vi "PitchCalc.vi"(10 "Previous Pitch Value":dbl, 11 "Pitch Control":dbl) -> (2 "New Pitch Value":dbl, 3 "Adjustment to be made":dbl)   [LabVIEW 2014, in "lv-attitudecontrol.lvlib"]
uses:
  lv-attitudecontrol.lvlib
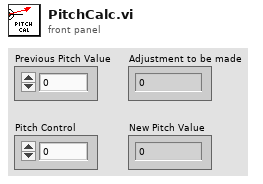
[diagram p1: front panel]
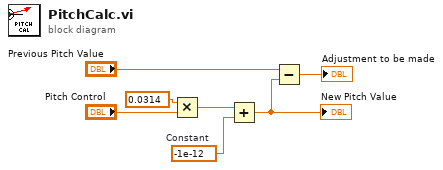
[diagram p0: block diagram]
diagram:
  w1 = -1e-12  # Constant
  n1 = Multiply(x=0.0314, y="Pitch Control") -> (x*y=w5:dbl)
  n2 = Add(x=w5, y=w1) -> (x+y=w7:dbl)
  "New Pitch Value" <- w7
  n3 = Subtract(x="Previous Pitch Value", y=w7) -> (x-y=→"Adjustment to be made":dbl)
